vi "Send Direct Unlock Publication.vi"(6 "Publisher ID":string, 7 "Message Priority (Normal)":T1=enum."Normal", 8 "error in (no error)":errorcluster, 9 "Datum Type":variant, 10 "Datum Name":string, 11 "Mediator Enqeuer":refnum<class "Message Enqueuer.lvclass">) -> (0 "error out":errorcluster, 3 "Mediator Enqueuer out":refnum<class "Message Enqueuer.lvclass">)   [LabVIEW 2017, in "IMediator.lvlib" / "Unlock Publication Msg.lvclass"]
doc: "This VI sends a message to the Mediator directly (as in cases where the ViewModel might want to publish a general system datum--like status--for Views to observe). Only the Controller should have a direct queue to the Mediator, so it is highly unlikely that any non-Controller class would call this VI.\n\n<License>\nCopyright © 2017 Composed Systems, LLC | All rights reserved\nwww.composed.io\n\nAuthor: Ethan Stern <ethan.stern@composed.io>\n\nThis software is provided \"AS IS\" WITHOUT WARRANTIES, either express or implied, AND IS FOR EDUCATIONAL PURPOSES ONLY.\n</License>"
uses:
  Unlock Publication Msg.lvclass
  <vilib>/ActorFramework/Message Enqueuer/Message Enqueuer.lvclass
  <vilib>/ActorFramework/Message Enqueuer/Message Priority.ctl
  C:/Program Files (x86)/National Instruments/LabVIEW 2017/vi.lib/ActorFramework/Message/Message.lvclass
  Unlock Publication Msg.lvclass/Unlock Publication Msg.ctl
  <vilib>/ActorFramework/Message Enqueuer/Message Enqueuer.lvclass/Message Enqueuer.ctl
  <vilib>/ActorFramework/Message Priority Queue/Priority Enqueue.vi
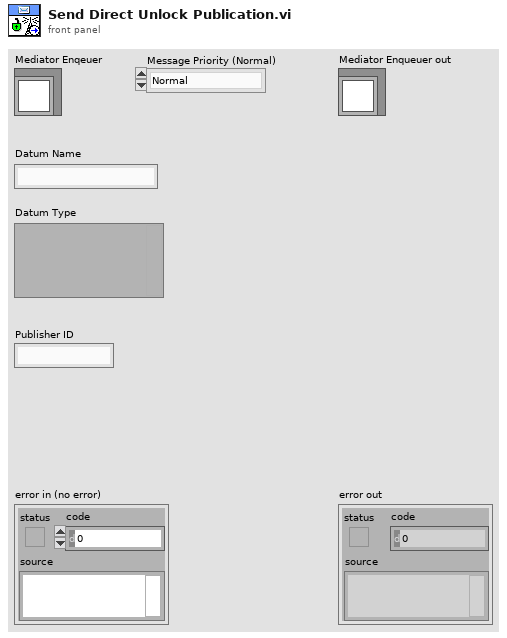
[diagram p1: front panel]
types:
  T1 = typedef "Actor Framework.lvlib/Message Enqueuer.lvclass/Message Priority.ctl" = enum16{"Low", "Normal", "High"}
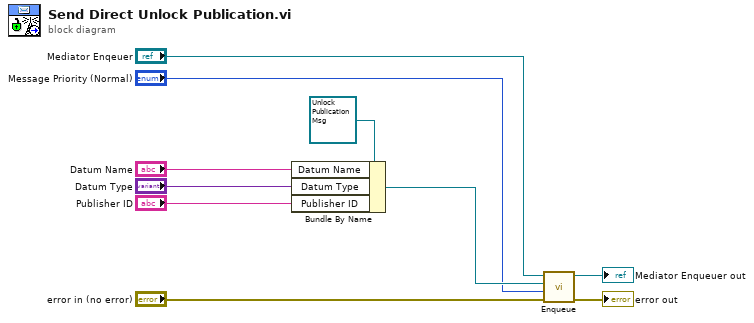
[diagram p0: block diagram]
diagram:
  n1 = Bundle By Name(cluster=refnum<class "Unlock Publication Msg.lvclass"> refnum ("Publish Message"), "Datum Name"="Datum Name", "Datum Type"="Datum Type", "Publisher ID"="Publisher ID") -> (w5:refnum<class "Unlock Publication Msg.lvclass">)
  n2 = call <vilib>:"Enqueue.vi"("error in (no error)"="error in (no error)", "Message Priority (Normal)"="Message Priority (Normal)", "Message"=w5, "Message Enqueuer in"="Mediator Enqeuer") -> ("error out"=→"error out":errorcluster, "Message Enqueuer out"=→"Mediator Enqueuer out":refnum<class "Message Enqueuer.lvclass">)  [unwired: 6 in]
